vi "Adv_ReadLightFieldProperty.vi"(8 "error in (no error)":errorcluster, 10 "setting":string, 11 "LightField Automation in":refnum<class "LightField Automation.lvclass">) -> (0 "error out":errorcluster, 2 "value":refnum<k24>, 3 "LightField Automation out":refnum<class "LightField Automation.lvclass">)   [LabVIEW 2015, in "LightField Automation.lvclass"]
uses:
  LightField Automation.lvclass
  C:/Program Files/Princeton Instruments/LightField/AddInViews/PrincetonInstruments.LightFieldViewV3.dll
  Program Files/Princeton Instruments/LightField/AddInViews/PrincetonInstruments.LightFieldViewV3.dll
  <vilib>/Utility/error.llb/DialogType.ctl
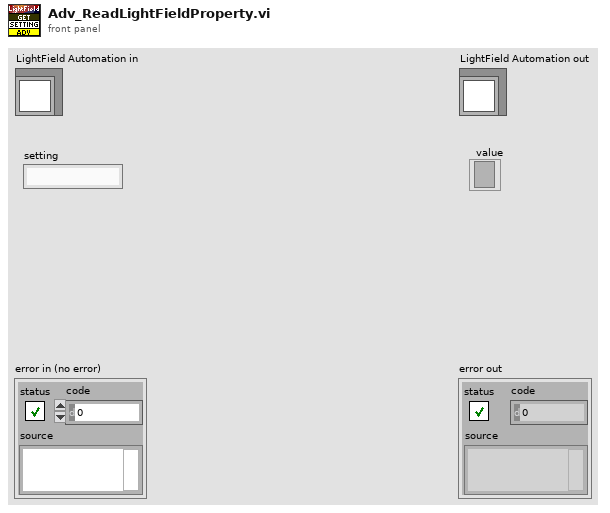
[diagram p1: front panel]
types:
  T1 = typedef "DialogType.ctl" = u16
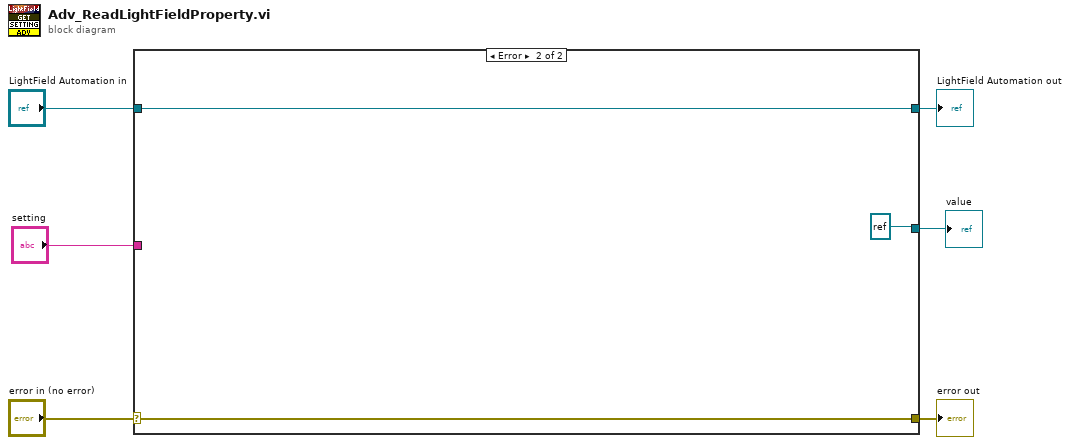
[diagram p0: block diagram]
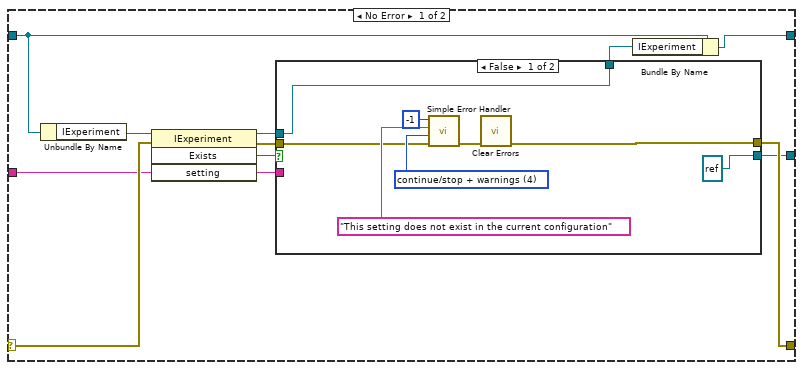
[diagram p2: hidden frame]
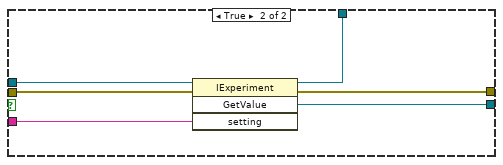
[diagram p3: hidden frame]
diagram:
  n1 = case shown="Error" "error in (no error)" {
    selector: "error in (no error)" -> [w15 w34]
    tunnel: [w17 w34] -> w5
    tunnel: [w8 w33] -> w3
    tunnel: "LightField Automation in" -> [w9 w33]
    tunnel: "setting" -> [w11 _]
    tunnel: [w10 refnum<k24> refnum ("GetValue")] -> w1
    frame No Error {
      n2 = Unbundle By Name(w9) -> ("IExperiment"=w16:refnum<k24>)
      n3 = invoke class="IExperiment" method="Exists"(reference=w16, error in=w15, "setting"=w11) -> (reference out=w13:refnum<k24>, error out=w12:errorcluster, "Exists"=w14:bool)  [unwired: 1 in, 1 out]
      n4 = case shown="False" w14 {
        tunnel: [w22 w26] -> w17
        tunnel: w13 -> [w19 w31]
        tunnel: w12 -> [w20 w30]
        tunnel: w11 -> [_ w29]
        tunnel: [refnum<k24> refnum ("GetValue") w28] -> w10
        tunnel: [w19 w27] -> w7
        frame False {
          w21 = T1 4 items=["no dialog", "OK message", "continue or stop message", "OK message + warnings", "continue/stop + warnings"] ("type of dialog (OK msg:1)")
          n5 = call <vilib>:"Simple Error Handler.vi"("error code (no error:0)"=-1, "error source (\" \")"="This setting does not exist in the current configuration" ("source"), "type of dialog (OK msg:1)"=w21, "error in (no error)"=w20) -> ("error out"=w23:errorcluster)  [unwired: 1 in, 4 out]
          n6 = call <vilib>:"Clear Errors.vi"("error in (no error)"=w23) -> ("error out"=w22:errorcluster)  [unwired: 5 in, 1 out]
        }
        frame True {
          n7 = invoke class="IExperiment" method="GetValue"(reference=w31, error in=w30, "setting"=w29) -> (reference out=w27:refnum<k24>, error out=w26:errorcluster, "GetValue"=w28:refnum<k24>)  [unwired: 1 in, 1 out]
        }
      }
      n8 = Bundle By Name(cluster=w9, "IExperiment"=w7) -> (w8:refnum<class "LightField Automation.lvclass">)
    }
    frame Error {
    }
  }
  "error out" <- w5
  "LightField Automation out" <- w3
  "value" <- w1
